vi "Add point to Waypoint Route.vi"(0 "Route Index":i32, 5 "MISSION_ITEM":T1={"target_system"=0, "target_component"=0, "sequence"=0, "frame"=enum."GLOBAL RELATIVE ALT", "command"=0, "current"=FALSE, "autocontinue"=FALSE, "param1"=0.0, "param2"=0.0, "param3"=0.0, "param4"=0.0, "Lat"=0.0, "Lon"=0.0, "Altitude (m)"=0.0}, 7 "Main Map DLL Ref":refnum<k24>, 9 "Main Map Control Reference":refnum<k24>, 11 "Error In":errorcluster) -> (15 "Error Out":errorcluster)   [LabVIEW 2014]
uses:
  C:/Robotic Systems/Products/Surveyor/Software/Ground Station/Data/Mapping DLL/GMap.NET.WindowsForms.dll
  Data/Mapping DLL/GMap.NET.WindowsForms.dll
  MAVLink/Controls/Mission Planning Controls/MAVLINK Mission Item.ctl
  MAVLink/Controls/MAVLINK Mav Frame.ctl
  C:/Robotic Systems/Products/Surveyor/Software/Ground Station/Data/Mapping DLL/GMap.NET.Core.dll
  Data/Mapping DLL/GMap.NET.Core.dll
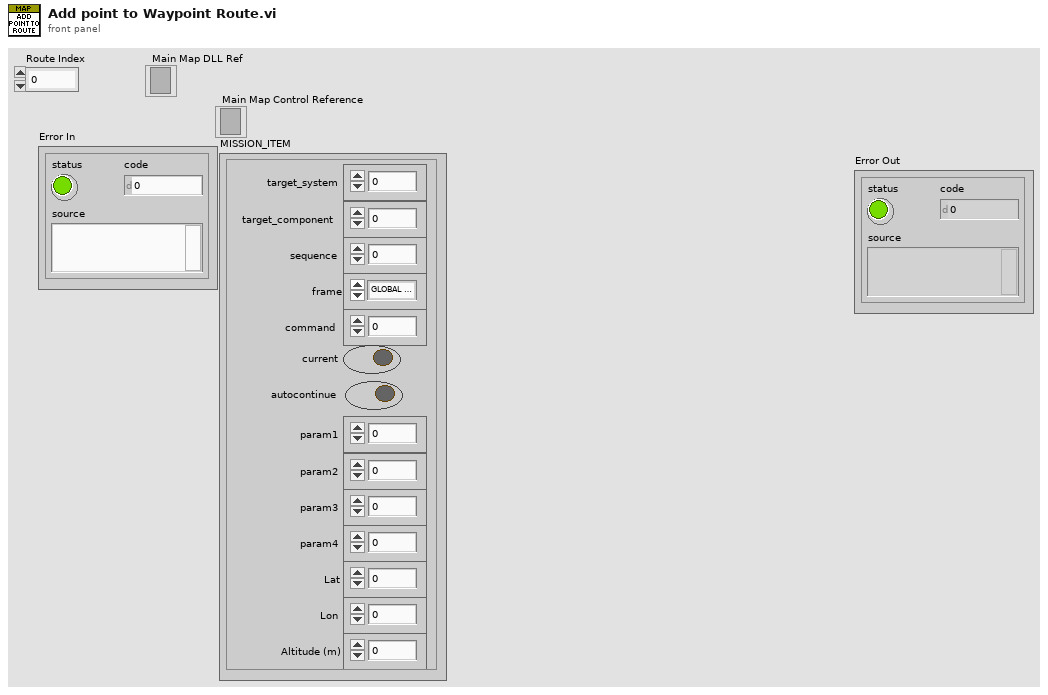
[diagram p1: front panel]
types:
  T1 = typedef "MAVLINK Mission Item.ctl" = cluster{"target_system":u8, "target_component":u8, "sequence":u16, "frame":T2, "command":u16, "current":bool, "autocontinue":bool, "param1":sgl, "param2":sgl, "param3":sgl, "param4":sgl, "Lat":sgl, "Lon":sgl, "Altitude (m)":sgl}
  T2 = typedef "MAVLINK Mav Frame.ctl" = enum8{"GLOBAL", "LOCAL NED", "MISSION", "GLOBAL RELATIVE ALT", "LOCAL ENU", "GLOBAL INT", "GLOBAL RELATIVE ALT INT", "LOCAL OFFSET NED", "BODY NED", "BODY OFFSET NED", "GLOBAL TERRAIN ALT", "GLOBAL TERRAIN ALT INT"}
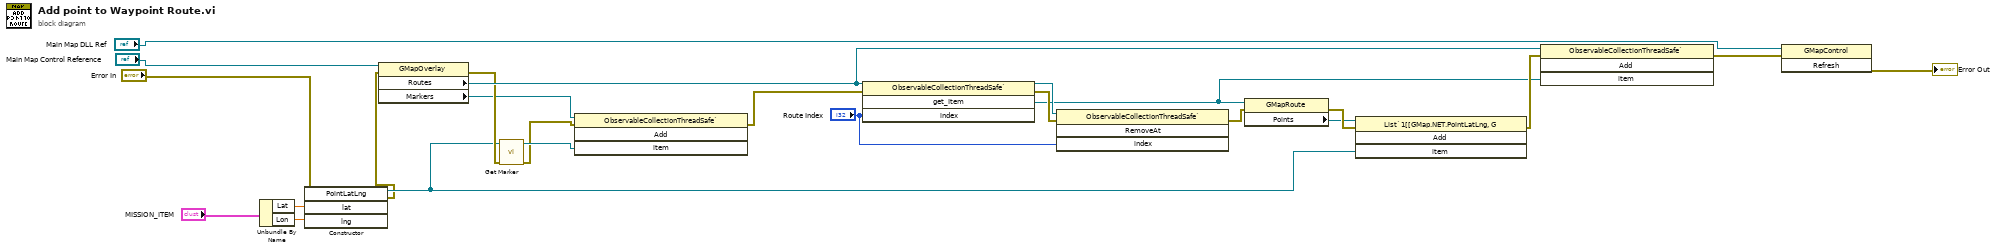
[diagram p0: block diagram]
diagram:
  n1 = Unbundle By Name("MISSION_ITEM") -> ("Lat"=w10:sgl, "Lon"=w9:sgl)
  n2 = constructor class="PointLatLng"(error in="Error In", "lat"=w10, "lng"=w9) -> (reference out=w6:refnum<k24>, error out=w1:errorcluster)  [unwired: 2 in, 3 out]
  n3 = property class="GMapOverlay"(reference="Main Map Control Reference", error in=w1) -> (error out=w7:errorcluster, "Routes"=w14:refnum<k24>, "Markers"=w3:refnum<k24>)  [unwired: 1 out]
  n4 = call "Get Marker.vi"("Error In"=w7, "Point"=w6) -> ("error out"=w5:errorcluster, "new reference"=w8:refnum<k24>)  [unwired: 8 in]
  n5 = invoke class="ObservableCollectionThreadSafe`" method="Add"(reference=w3, error in=w5, "item"=w8) -> (error out=w4:errorcluster)  [unwired: 1 in, 3 out]
  n6 = invoke class="ObservableCollectionThreadSafe`" method="get_Item"(reference=w14, error in=w4, "index"="Route Index") -> (reference out=w22:refnum<k24>, error out=w24:errorcluster, "get_Item"=w17:refnum<k24>)  [unwired: 1 in, 1 out]
  n7 = invoke class="ObservableCollectionThreadSafe`" method="RemoveAt"(reference=w22, error in=w24, "index"="Route Index") -> (error out=w21:errorcluster)  [unwired: 1 in, 3 out]
  n8 = property class="GMapRoute"(reference=w17, error in=w21) -> (error out=w20:errorcluster, "Points"=w18:refnum<k24>)  [unwired: 1 out]
  n9 = invoke class="List`1[[GMap.NET.PointLatLng, G" method="Add"(reference=w18, error in=w20, "item"=w6) -> (error out=w19:errorcluster)  [unwired: 1 in, 3 out]
  n10 = invoke class="ObservableCollectionThreadSafe`" method="Add"(reference=w14, error in=w19, "item"=w17) -> (error out=w16:errorcluster)  [unwired: 1 in, 3 out]
  n11 = invoke class="GMapControl" method="Refresh"(reference="Main Map DLL Ref", error in=w16) -> (error out=→"Error Out":errorcluster)  [unwired: 1 in, 2 out]
